vi "Selftest Device Core.vi"(8 "error in (no error)":errorcluster, 11 "CS++DeviceActor in":refnum<class "CS++DeviceActor.lvclass">) -> (0 "error out":errorcluster, 1 "Self-Test Result Message":string, 2 "Self-Test Result Code":i32, 3 "CS++DeviceActor out":refnum<class "CS++DeviceActor.lvclass">)   [LabVIEW 2015, in "CS++DeviceActor.lvlib" / "CS++DeviceActor.lvclass"]
doc: "Perform selftest of device."
uses:
  CS++DeviceActor.lvclass
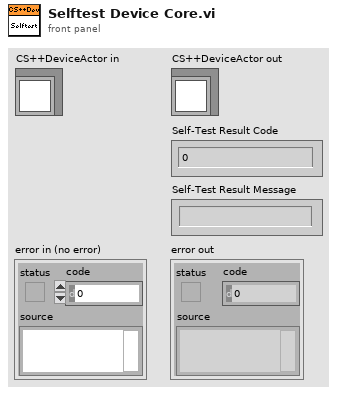
[diagram p1: front panel]
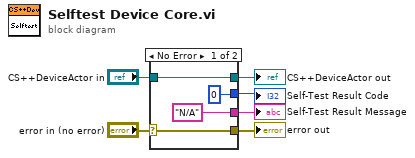
[diagram p0: block diagram]
diagram:
  n1 = case shown="No Error" "error in (no error)" {
    selector: "error in (no error)" -> [w9 w12]
    tunnel: [w9 w12] -> w5
    tunnel: [w10 w11] -> w3
    tunnel: "CS++DeviceActor in" -> [w10 w11]
    tunnel: [0 _] -> w1
    tunnel: ["N/A" _] -> w2
    frame No Error {
    }
    frame Error {
    }
  }
  "error out" <- w5
  "CS++DeviceActor out" <- w3
  "Self-Test Result Code" <- w1
  "Self-Test Result Message" <- w2
